vi "Configuration Tool Main.vi"() -> ()   [LabVIEW 2015, in "Configuration Tool.lvlib"]
doc: "This is the main VI for the configuration editor.Copyright 2017 National Instruments Corporation\n\nLicensed under the Apache License, Version 2.0 (the \"License\"); you may not use this file except in compliance with the License. You may obtain a copy of the License at http://www.apache.org/licenses/LICENSE-2.0\nUnless required by applicable law or agreed to in writing, software distributed under the License is distributed on an \"AS IS\" BASIS, WITHOUT WARRANTIES OR CONDITIONS OF ANY KIND, either express or implied. See the License for the specific language governing permissions and limitations under the License."
uses:
  Configuration Tool.lvlib
  Controls/StateCluster.ctl
  <vilib>/NI/Configuration Framework/Repository/NISE_CEF_Repository.lvclass
  <vilib>/NI/Configuration Framework/Node/NodeRef.ctl
  <vilib>/NI/Configuration Framework/Node/NISE_CEF_Node.lvclass
  <vilib>/NI/Configuration Framework/Node/StandardEvents.ctl
  <vilib>/NI/Configuration Framework/Node/UserEventRef.ctl
  <vilib>/NI/Configuration Framework/Controls/EventCluster.ctl
  <vilib>/NI/Configuration Framework/Node/NodeChangeEvent.ctl
  <vilib>/NI/Configuration Framework/Node/CacheState.ctl
  <vilib>/NI/Configuration Framework/Node/RefreshUIEvent.ctl
  <vilib>/NI/Configuration Framework/Node/StopEvent.ctl
  <vilib>/NI/Configuration Framework/glyph manager/glyph manager.ctl
  <vilib>/picture/picture.llb/imagedata.ctl
  Controls/StepClassLibrary.ctl
  Prototype/classes/Step/Config/Step Config.lvclass
  Controls/AddMessage.ctl
  Controls/MoveMessage.ctl
  <vilib>/Utility/error.llb/DialogType.ctl
  Classes/SequenceNode/SequenceNode.lvclass
  Classes/SequenceRepo/SequenceRepo.lvclass
  <vilib>/Utility/sysdir.llb/System Directory Type.ctl
  Classes/StepNode/StepNode.lvclass
  <vilib>/NI/AMC/Read Termination Message.vi
  <vilib>/NI/AMC/Create Single Message.vi
  <vilib>/NI/AMC/Update Message Routing Info.vi
  <vilib>/NI/AMC/Send Message.vi
  <vilib>/NI/AMC/Globals.vi
  <vilib>/NI/AMC/AMC.lvlib
  <vilib>/NI/Configuration Framework/NISE_CEF_TreeControl.lvlib
  <vilib>/NI/Configuration Framework/glyph manager/glyph manager.lvlib
panel:
  in  "View":string(tree)
  in  "Exit":bool
  # "Configurator"
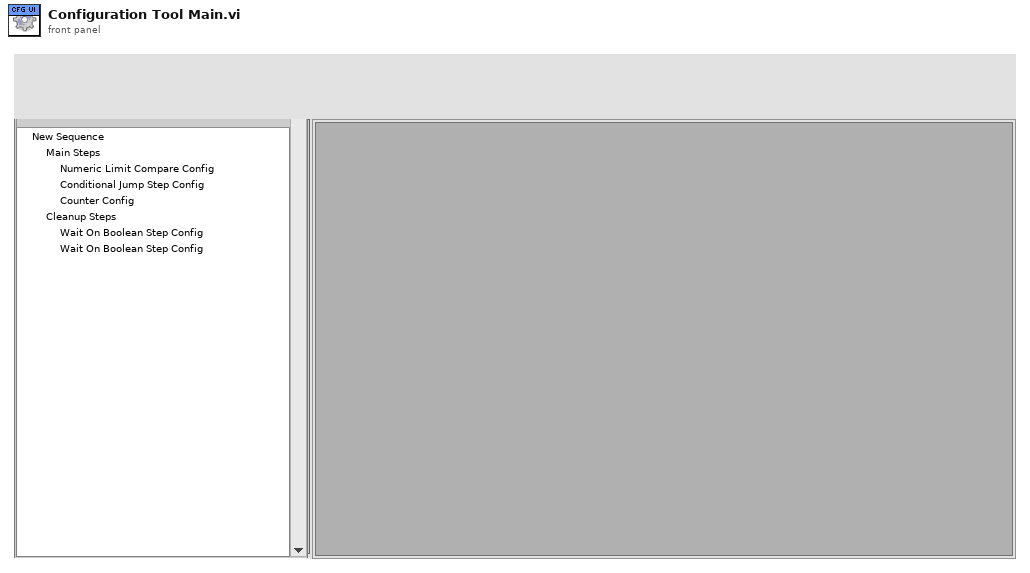
[diagram p1: front panel]
types:
  T1 = typedef "Configuration Tool.lvlib/StateCluster.ctl" = cluster{"repository":refnum<class "NISE_CEF_Repository.lvclass">, "root":T2, "unsaved changes":bool, "current path":path, "standard events":T3, "classes path":path, "glyph manager":T9, "Step Class Library":T11}
  T2 = typedef "NISE_CEF_Node.lvclass/NodeRef.ctl" = refnum<data-value>
  T3 = typedef "NISE_CEF_Node.lvclass/StandardEvents.ctl" = cluster{"user event":T4, "node change":T5, "cache state":T6, "refresh UI":T7, "stop event":T8}
  T4 = typedef "NISE_CEF_Node.lvclass/UserEventRef.ctl" = refnum<user-event>
  T5 = typedef "NISE_CEF_Node.lvclass/NodeChangeEvent.ctl" = refnum<user-event>
  T6 = typedef "NISE_CEF_Node.lvclass/CacheState.ctl" = refnum<user-event>
  T7 = typedef "NISE_CEF_Node.lvclass/RefreshUIEvent.ctl" = refnum<user-event>
  T8 = typedef "NISE_CEF_Node.lvclass/StopEvent.ctl" = refnum<user-event>
  T9 = typedef "glyph manager.lvlib/glyph manager.ctl" = cluster{"search paths":path[], "glyph map":variant, "base glyphs":T10[], "desired overlays":string[]}
  T10 = typedef "imagedata.ctl" = cluster{"image type":i32, "image depth":i32, "image":u8[], "mask":u8[], "colors":u32[], "Rectangle":cluster{"left":i16, "top":i16, "right":i16, "bottom":i16}}
  T11 = typedef "StepClassLibrary.ctl" = cluster{"Step Types":string[], "Step Config Classes":refnum<class "Step Config.lvclass">[]}
  T12 = typedef "AMC.lvlib/Message Queue.ctl" = refnum<queue>
  T13 = typedef "Configuration Tool.lvlib/AddMessage.ctl" = cluster{"node type":string, "to add to":string}
  T14 = typedef "Configuration Tool.lvlib/MoveMessage.ctl" = cluster{"node ref":T2, "new parent":T2, "Index":i32}
  T15 = typedef "Configuration Tool.lvlib/FilePaths.ctl" = cluster{"glyphs":path, "classes":path}
  T16 = typedef "DialogType.ctl" = u16
  T17 = typedef "System Directory Type.ctl" = i32
  T18 = typedef "NISE_CEF_Node.lvclass/Summary.ctl" = cluster{"ID":string, "parent ID":string, "node type":string, "text":string, "additional text":string, "glyph":string, "depth":i32, "glyph overlay":string}
  T19 = typedef "LVPoint32TypeDef.ctl" = cluster{"Horizontal":i32, "Vertical":i32}
  T20 = cluster{"data name":string, "drag data":variant}[]
  T21 = typedef "NISE_CEF_Node.lvclass/NodeMenuOptions.ctl" = cluster{"removable":bool, "movable":bool, "duplicate":bool}
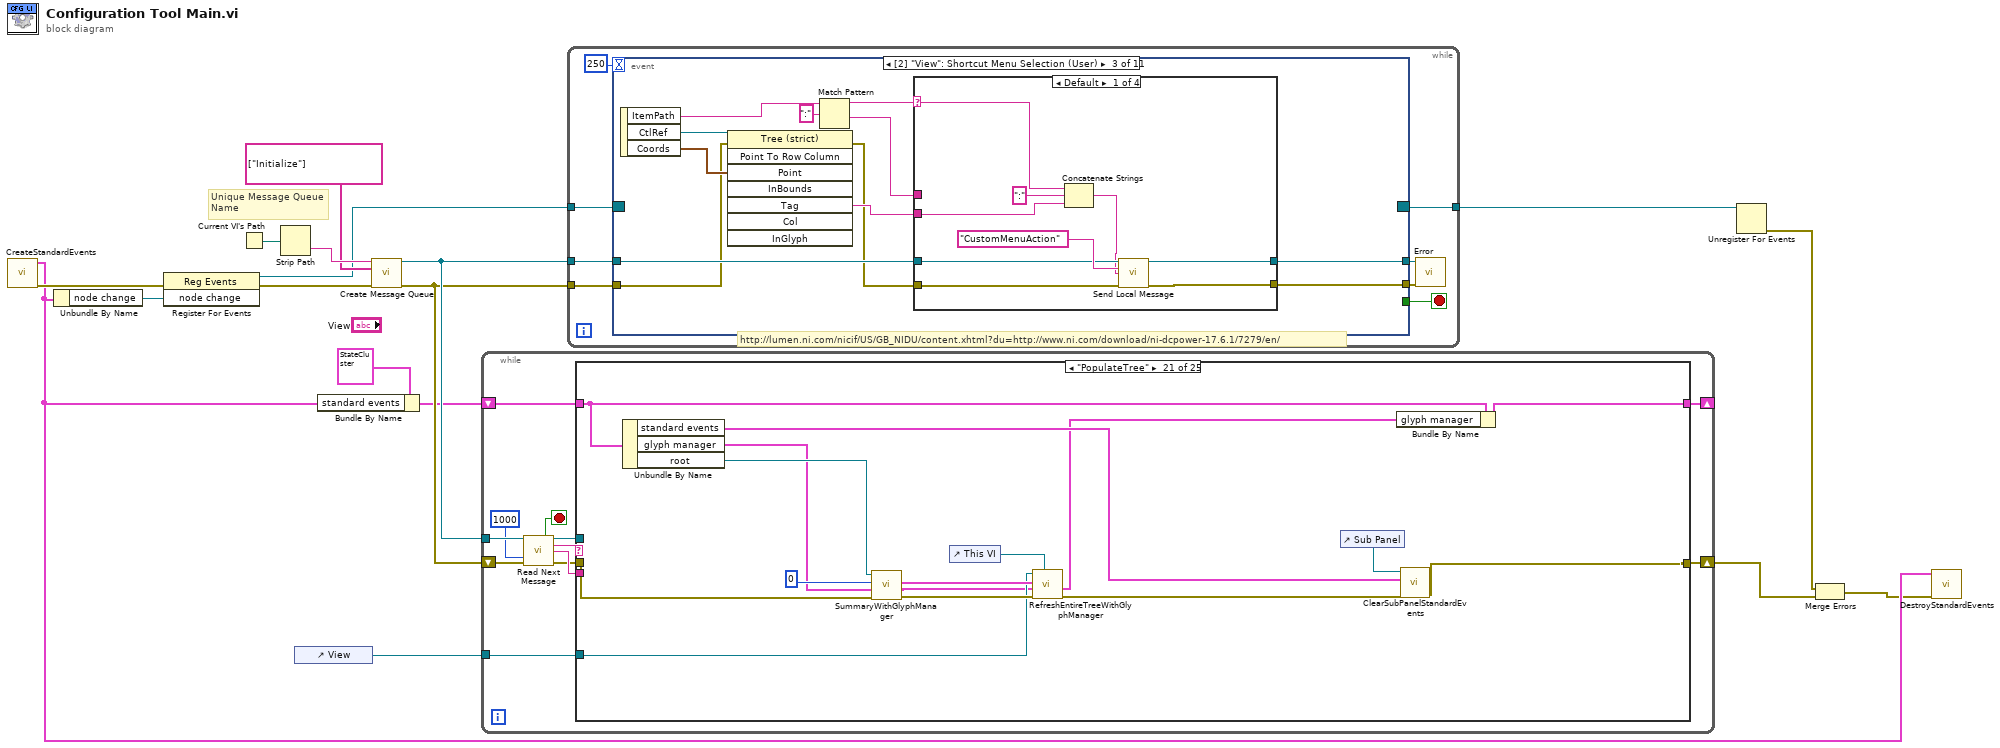
[diagram p0: block diagram]
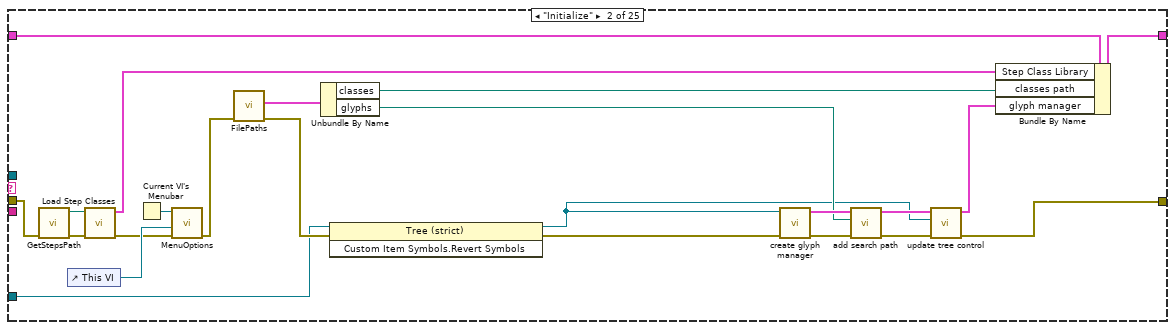
[diagram p3: hidden frame]
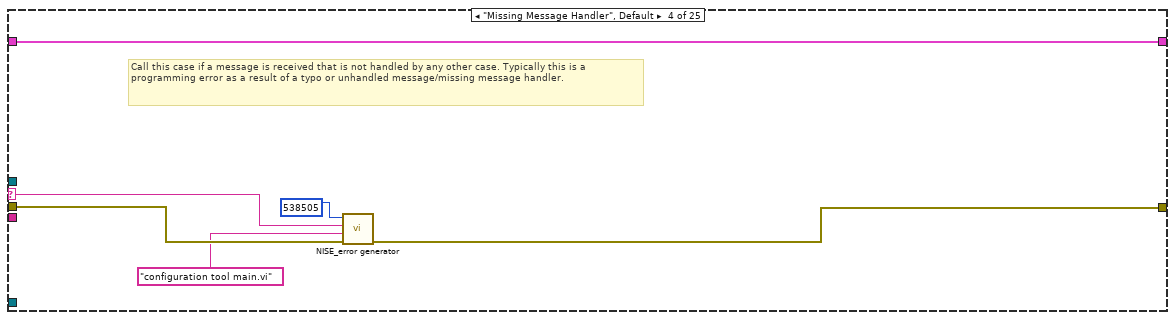
[diagram p5: hidden frame]
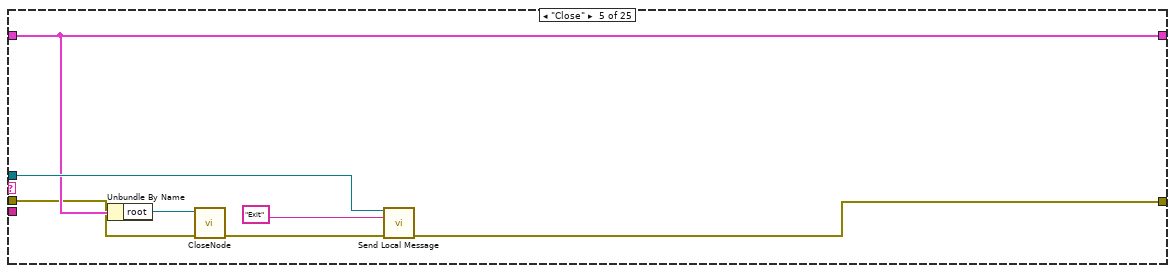
[diagram p6: hidden frame]
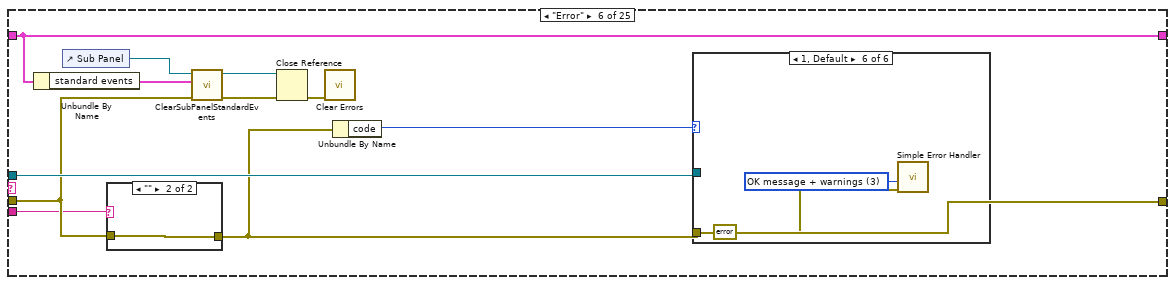
[diagram p7: hidden frame]
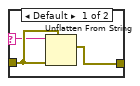
[diagram p8: hidden frame]
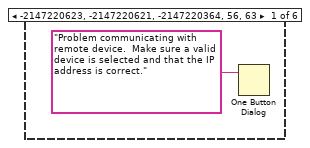
[diagram p9: hidden frame]
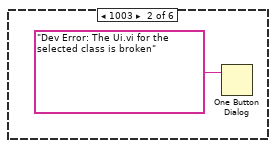
[diagram p10: hidden frame]
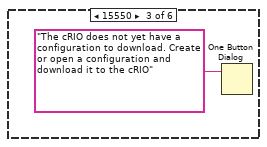
[diagram p11: hidden frame]
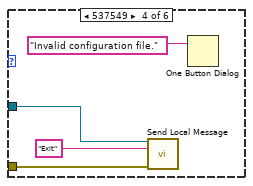
[diagram p12: hidden frame]
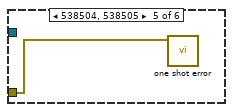
[diagram p13: hidden frame]
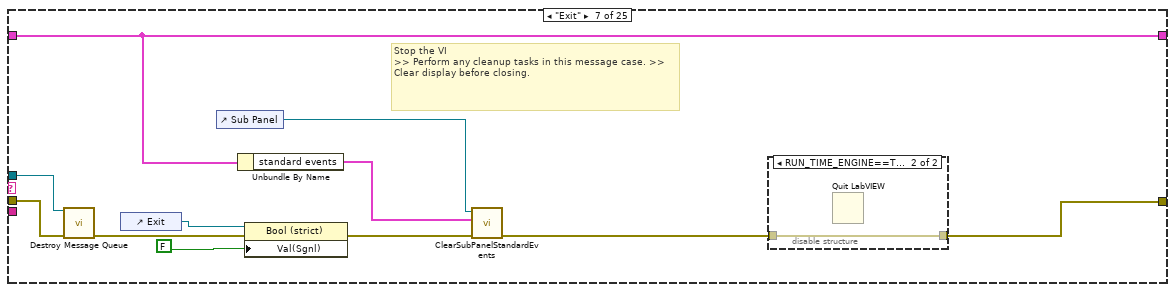
[diagram p14: hidden frame]
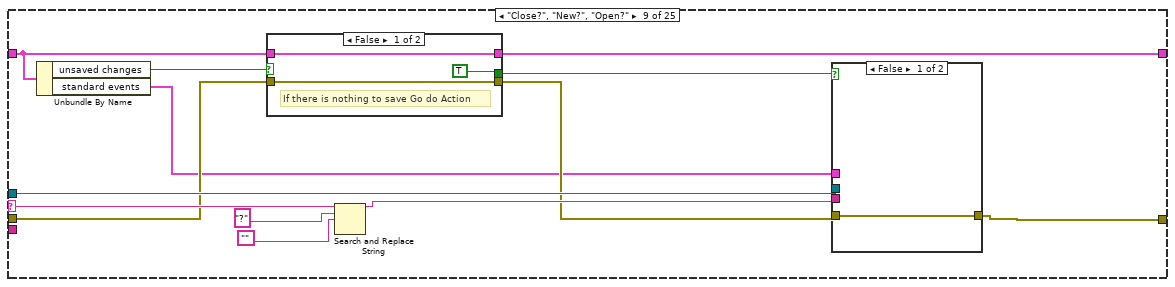
[diagram p17: hidden frame]
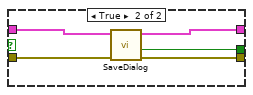
[diagram p18: hidden frame]
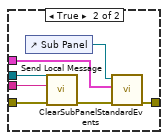
[diagram p19: hidden frame]
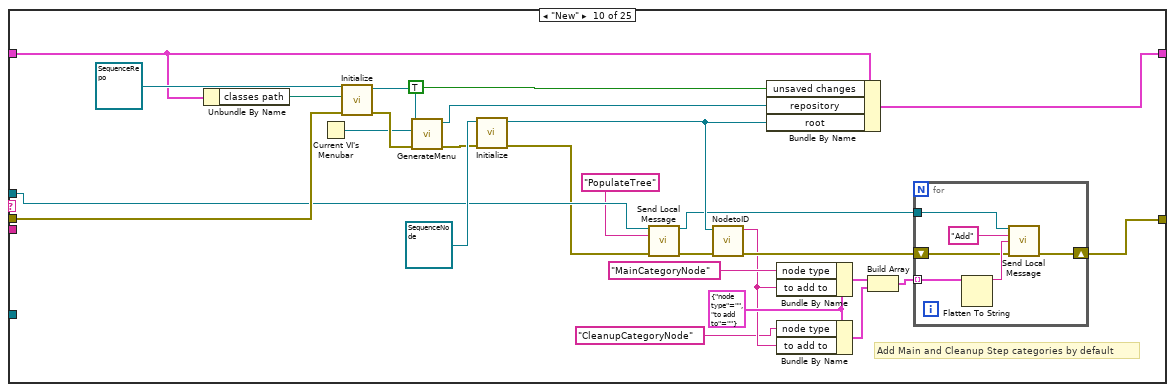
[diagram p20: hidden frame]
diagram:
  # "http://lumen.ni.com/nicif/US/GB_NIDU/content.xhtml?du=http://www.ni.com/download/ni-dcpower-17.6.1/7279/en/"
  # "Unique Message Queue Name"
  n1 = call <vilib>:"CreateStandardEvents.vi"() -> ("error out"=w12:errorcluster, "standard events"=w6:T3)  [unwired: 10 in]
  n2 = Unbundle By Name(w6) -> ("node change"=w11:T5)
  n3 = register-events(error in=w12, w11) -> (reference out=w5:refnum<event-registration>, error out=w10:errorcluster)  [unwired: 1 in]
  n4 = Current VI's Path() -> (path=w16:path)
  n5 = Strip Path(path=w16) -> (name=w17:string)  [unwired: 1 out]
  n6 = control-ref of="View"() -> (w4:refnum<vi>)
  n7 = Bundle By Name(cluster=T1 {"repository"=refnum, "root"=refnum, "unsaved changes"=FALSE, "current path"=path "", "standard events"={"user event"=refnum, "node change"=refnum, "cache state"=refnum, "refresh UI"=refnum, "stop event"=refnum}, "classes path"=path "", "glyph manager"={"search paths"=[], "glyph map"=variant, "base glyphs"=[], "desired overlays"=[]}, "Step Class Library"={"Step Types"=[], "Step Config Classes"=[]}}, "standard events"=w6) -> (w8:T1)
  n8 = call <vilib>:"Create Message Queue.vi"("message queue name"=w17, "initial message names"=string[] ["Initialize"], "error in"=w10) -> ("message queue out"=w14:T12, "error out"=w13:errorcluster)  [unwired: 11 in]
  n9 = while "Message Processor" {
    shift-right: [w25] -> w7
    shift-left: w13 -> [w24]
    tunnel: w14 -> [w23]
    shift-right: [w21] -> _
    shift-left: w8 -> [w20]
    tunnel: w4 -> [w18]
    stop <- w29 stop-if-true
    n10 = call <vilib>:"Read Next Message.vi"("message queue in"=w23, "timeout (1 ms)"=1000, "error in"=w24) -> ("exit process?"=w29:bool, "message queue out"=w19:T12, "message name"=w28:string, "message value"=w27:string, "error out"=w26:errorcluster)  [unwired: 5 in, 3 out]
    n11 = case shown="\"PopulateTree\"" w28 {
      selector: w28 -> [_ _ _ w58 _ _ _ _ w119 _ _ _ _ _ _ _ _ w352 _ _ _ _ _ _ _]
      tunnel: w27 -> [_ _ _ _ _ w71 _ _ _ _ _ _ _ w253 _ w302 w330 w350 w402 w426 _ _ w466 w487 w494]
      tunnel: w26 -> [w31 w32 w56 w61 w64 w74 w106 w110 w112 w160 w179 w219 w245 w260 w273 w294 w329 w355 w404 w425 w447 w456 w465 w485 w495]
      tunnel: [w31 w43 w56 w59 w68 errorcluster {"status"=FALSE, "code"=0, "source"=""} ("error out") w98 w110 w123 w153 w175 w223 w247 w257 w273 w296 w333 w358 w406 w422 w441 w452 w462 w480 w493] -> w25
      tunnel: [w30 w50 w55 w62 w66 w78 w97 w109 w114 w166 w180 w226 w246 w254 w272 w289 w326 w359 w405 w427 w438 w455 w460 w488 w490] -> w21
      tunnel: w20 -> [w30 w51 w55 w62 w66 w78 w97 w109 w115 w162 w181 w221 w244 w255 w272 w292 w327 w359 w397 w427 w450 w455 w460 w488 w496]
      tunnel: w19 -> [_ _ _ _ w67 w81 w105 _ w122 w151 w177 w222 _ w256 _ _ _ w353 _ _ _ _ w461 w479 w492]
      tunnel: w18 -> [_ w37 _ _ _ _ _ _ _ _ _ _ _ _ _ w290 w322 w347 w399 w420 w439 _ _ _ _]
      frame "------------Generic Operations------------" {
        # "Dummy case to add a seperation in the Case Structure menu"
      }
      frame "Initialize" {
        n12 = call "GetStepsPath.vi"("error in (no error)"=w32) -> ("error out"=w33:errorcluster, "Steps Folder Path"=w34:path)  [unwired: 9 in]
        n13 = control-ref of="This VI"() -> (w54:refnum<vi>)
        n14 = call "Load Step Classes.vi"("error in (no error)"=w33, "Step Classes Folder Path"=w34) -> ("error out"=w36:errorcluster, "Step Class Library"=w35:T11)  [unwired: 8 in]
        n15 = Current VI's Menubar() -> (w53:refnum<k9>)
        n16 = call "MenuOptions.vi"("error in"=w36, "VI ref"=w54, "menu ref in"=w53) -> ("error out"=w49:errorcluster)  [unwired: 7 in, 1 out]
        n17 = call "FilePaths.vi"("error in"=w49) -> ("error out"=w40:errorcluster, "paths"=w52:T15)  [unwired: 9 in]
        n18 = Unbundle By Name(w52) -> ("classes"=w48:path, "glyphs"=w42:path)
        n19 = invoke class="Tree (strict)" method="Custom Item Symbols.Revert Symbols"(reference=w37, error in=w40) -> (reference out=w38:refnum<vi>, error out=w39:errorcluster)  [unwired: 1 in, 1 out]
        n20 = call <vilib>:"create glyph manager.vi"("error in"=w39, "tree ref (for default symbols)"=w38) -> ("error out"=w47:errorcluster, "glyph manager"=w46:T9)  [unwired: 8 in]
        n21 = call <vilib>:"add search path.vi"("error in"=w47, "search path"=w42, "glyph manager in"=w46) -> ("error out"=w45:errorcluster, "glyph manager out"=w44:T9)  [unwired: 7 in]
        n22 = call <vilib>:"update tree control.vi"("error in"=w45, "tree reference"=w38, "glyph manager in"=w44) -> ("error out"=w43:errorcluster, "glyph manager out"=w41:T9)  [unwired: 7 in]
        n23 = Bundle By Name(cluster=w51, "Step Class Library"=w35, "classes path"=w48, "glyph manager"=w41) -> (w50:T1)
      }
      frame "", "Idle" {
      }
      frame "Missing Message Handler", Default {
        # "Call this case if a message is received that is not handled by any other case. Typically this is a programming error as a result of a typo or unhandled message/missing message handler."
        n24 = call <vilib>:"NISE_error generator.vi"("error in"=w61, "source"="configuration tool main.vi", "append error message"=w58, "error code (0)"=538505) -> ("error out"=w59:errorcluster)  [unwired: 5 in]
      }
      frame "Close" {
        n25 = Unbundle By Name(w66) -> ("root"=w65:T2)
        n26 = call <vilib>:"CloseNode.vi"("error in"=w64, "node ref"=w65) -> ("error out"=w63:errorcluster)  [unwired: 9 in]
        n27 = call <vilib>:"Send Local Message.vi"("message queue in"=w67, "message name"="Exit", "error in"=w63) -> ("error out"=w68:errorcluster)  [unwired: 10 in, 2 out]
      }
      frame "Error" {
        n28 = Unbundle By Name(w78) -> ("standard events"=w70:T3)
        n29 = control-ref of="Sub Panel"() -> (w77:refnum<vi>)
        n30 = case shown="\"\"" w71 {
          selector: w71 -> [w83 _]
          tunnel: w74 -> [w84 w85]
          tunnel: [w82 w85] -> w73
          frame Default {
            n31 = Unflatten From String(type=w84, binary string=w83, error in (no error)=w84) -> (value=w82:errorcluster)  [unwired: 2 in, 2 out]
          }
          frame "" {
          }
        }
        n32 = call <vilib>:"ClearSubPanelStandardEvents.vi"("error in"=w74, "standard events"=w70, "sub panel ref in"=w77) -> ("error out"=w76:errorcluster, "sub panel ref out"=w75:refnum<vi>)  [unwired: 7 in]
        n33 = Close Reference(reference=w75, error in (no error)=w76) -> (error out=w72:errorcluster)
        n34 = call <vilib>:"Clear Errors.vi"("error in (no error)"=w72) -> ()  [unwired: 5 in, 2 out]
        n35 = Unbundle By Name(w73) -> ("code"=w79:i32)
        n36 = case shown="1, Default" w79 {
          tunnel: w81 -> [_ _ _ w91 _ _]
          tunnel: w73 -> [_ _ _ w90 w93 w95]
          frame -2147220623, -2147220621, -2147220364, 56, 63 {
            n37 = One Button Dialog(message="Problem communicating with remote device.  Make sure a valid device is selected and that the IP address is correct.") -> ()  [unwired: 1 in, 1 out]
          }
          frame 1003 {
            n38 = One Button Dialog(message="Dev Error: The Ui.vi for the selected class is broken") -> ()  [unwired: 1 in, 1 out]
          }
          frame 15550 {
            n39 = One Button Dialog(message="The cRIO does not yet have a configuration to download. Create or open a configuration and download it to the cRIO") -> ()  [unwired: 1 in, 1 out]
          }
          frame 537549 {
            n40 = call <vilib>:"Send Local Message.vi"("message queue in"=w91, "message name"="Exit", "error in"=w90) -> ()  [unwired: 10 in, 3 out]
            n41 = One Button Dialog(message="Invalid configuration file.") -> ()  [unwired: 1 in, 1 out]
          }
          frame 538504, 538505 {
            n42 = call <vilib>:"one shot error.vi"("error in"=w93) -> ()  [unwired: 11 in]
          }
          frame 1, Default {
            w94 = T16 3 items=["no dialog", "OK message", "continue or stop message", "OK message + warnings", "continue/stop + warnings"] ("type of dialog (OK msg:1)")
            n43 = call <vilib>:"Simple Error Handler.vi"("type of dialog (OK msg:1)"=w94, "error in (no error)"=w95) -> ()  [unwired: 8 out]
          }
        }
      }
      frame "Exit" {
        # "Stop the VI                                                                             >> Perform any cleanup tasks in this message case. >> Clear display before closing."
        n44 = call <vilib>:"Destroy Message Queue.vi"("message queue in"=w105, "error in"=w106) -> ("error out"=w102:errorcluster)  [unwired: 11 in, 2 out]
        n45 = control-ref of="Exit"() -> (w104:refnum<vi>)
        n46 = control-ref of="Sub Panel"() -> (w101:refnum<vi>)
        n47 = Unbundle By Name(w97) -> ("standard events"=w96:T3)
        n48 = property class="Bool (strict)"(reference=w104, error in=w102, "Val(Sgnl)"=FALSE ("Exit")) -> (error out=w100:errorcluster)  [unwired: 1 out]
        n49 = call <vilib>:"ClearSubPanelStandardEvents.vi"("error in"=w100, "standard events"=w96, "sub panel ref in"=w101) -> ("error out"=w99:errorcluster)  [unwired: 7 in, 1 out]
        n50 = disable-structure shown="RUN_TIME_ENGINE==True" {
          disable-tunnel: [w107 w108] -> w98
          disable-tunnel: w99 -> [w107 w108]
          frame condition #0 (active) {
          }
          frame condition #1 {
            n51 = Quit LabVIEW() -> ()  [unwired: 1 in]
          }
        }
      }
      frame "------------Menu Operations--------------" {
        # "Dummy case to add a seperation in the Case Structure menu"
      }
      frame "Close?", "New?", "Open?" {
        n52 = Unbundle By Name(w115) -> ("unsaved changes"=w117:bool, "standard events"=w111:T3)
        n53 = case shown="False" w117 {
          tunnel: [TRUE ("SaveFlag") w131] -> w116
          tunnel: w115 -> [w125 w130]
          tunnel: [w125 w129] -> w114
          tunnel: w112 -> [w124 w128]
          tunnel: [w124 w127] -> w113
          frame False {
            # "If there is nothing to save Go do Action"
          }
          frame True {
            n54 = call "SaveDialog.vi"("error in"=w128, "state in"=w130) -> ("error out"=w127:errorcluster, "new"=w131:bool, "state out"=w129:T1)  [unwired: 7 in]
          }
        }
        n55 = Search and Replace String(input string=w119, search string="?", replace string="") -> (result string=w118:string)  [unwired: 5 in, 3 out]
        n56 = case shown="False" w116 {
          tunnel: w113 -> [w132 w139]
          tunnel: [w132 w135] -> w123
          tunnel: w122 -> [_ w138]
          tunnel: w118 -> [_ w137]
          tunnel: w111 -> [_ w133]
          frame False {
          }
          frame True {
            n57 = control-ref of="Sub Panel"() -> (w134:refnum<vi>)
            n58 = call <vilib>:"Send Local Message.vi"("message queue in"=w138, "message name"=w137, "error in"=w139) -> ("error out"=w136:errorcluster)  [unwired: 10 in, 2 out]
            n59 = call <vilib>:"ClearSubPanelStandardEvents.vi"("error in"=w136, "standard events"=w133, "sub panel ref in"=w134) -> ("error out"=w135:errorcluster)  [unwired: 7 in, 1 out]
          }
        }
      }
      frame "New" {
        w143 = T13 {"node type"="", "to add to"=""} ("input cluster")
        # "Add Main and Cleanup Step categories by default"
        n60 = Unbundle By Name(w162) -> ("classes path"=w161:path)
        n61 = Current VI's Menubar() -> (w155:refnum<k9>)
        n62 = call-dynamic "Initialize.vi"("error in"=w160, "path"=w161, "repository in"=refnum<class "SequenceRepo.lvclass"> refnum ("cRIORepo.lvclass")) -> ("error out"=w159:errorcluster, "repository out"=w157:refnum<class "SequenceRepo.lvclass">)  [unwired: 7 in]
        n63 = call-dynamic "GenerateMenu.vi"("error in"=w159, "menu ref in"=w155, "NISE_CEF_Repository in"=w157) -> ("error out"=w158:errorcluster, "NISE_CEF_Repository out"=w156:refnum<class "SequenceRepo.lvclass">)  [unwired: 6 in, 1 out]
        n64 = call-dynamic "Initialize.vi"("error in"=w158, "SequenceNode in"=refnum<class "SequenceNode.lvclass"> refnum ("cRIO.lvclass")) -> ("error out"=w148:errorcluster, "data value reference"=w154:T2)  [unwired: 7 in, 1 out]
        n65 = call <vilib>:"Send Local Message.vi"("message queue in"=w151, "message name"="PopulateTree", "error in"=w148) -> ("message queue out"=w150:T12, "error out"=w147:errorcluster)  [unwired: 10 in, 1 out]
        n66 = call <vilib>:"NodetoID.vi"("error in"=w147, "node ref"=w154) -> ("error out"=w146:errorcluster, "ID"=w141:string)  [unwired: 8 in]
        n67 = Bundle By Name(cluster=w162, "unsaved changes"=TRUE ("SaveFlag"), "repository"=w156, "root"=w154) -> (w166:T1)
        n68 = Bundle By Name(cluster=w143, "node type"="MainCategoryNode", "to add to"=w141) -> (w144:T13)
        n69 = Bundle By Name(cluster=w143, "node type"="CleanupCategoryNode", "to add to"=w141) -> (w142:T13)
        n70 = Build Array(w144, w142) -> (w145:T13[])
        n71 = for {
          tunnel: w145 -> [w170] mode=indexing
          tunnel: w150 -> [w168]
          shift-right: [w172] -> w153
          shift-left: w146 -> [w167]
          n72 = Flatten To String(anything=w170) -> (data string=w169:string)  [unwired: 3 in, 2 out]
          n73 = call <vilib>:"Send Local Message.vi"("message queue in"=w168, "message name"="Add", "message value"=w169, "error in"=w167) -> ("error out"=w172:errorcluster)  [unwired: 9 in, 2 out]
        }
      }
      frame "Open" {
        w174 = T17 0 items=["User Home"=0, "User Desktop"=1, "User Documents"=2, "User Application Data"=3, "User Preferences"=4, "User Temporary"=5, "Public Documents"=6, "Public Application Data"=7, "Public Preferences"=8, "Public Cache"=13, "System Core Libraries"=9, "System Installed Libraries"=10, "Application Files"=11, "Boot Volume Root"=12] ("system directory type")
        n74 = call <vilib>:"Get System Directory.vi"("system directory type"=w174) -> ("system directory"=w173:path)  [unwired: 10 in]
        n75 = in-place {
          in-place-border: w179 -> [w187]
          in-place-border: [w186] -> w176
          in-place-border: w173 -> [w182]
          n76 = in-place-cluster #1(w181) -> ("current path"=w184:path, "repository"=w195:refnum<class "NISE_CEF_Repository.lvclass">, "root"=w191:T2)  [unwired: 1 out]
          n77 = call "FileDialog.vi"("error in"=w187, "start path"=w182) -> ("error out"=w188:errorcluster, "cancelled"=w189:bool, "selected path"=w185:path)  [unwired: 7 in]
          n78 = Compound Arithmetic op=OR(invert w189) -> (w190:bool)
          n79 = case shown="True" w190 {
            tunnel: w195 -> [w196 w208]
            tunnel: [w196 w206] -> w193
            tunnel: [w197 w204] -> w186
            tunnel: [w198 w203] -> w192
            tunnel: w185 -> [_ w201]
            tunnel: w188 -> [w197 w200]
            tunnel: w191 -> [w198 w199]
            frame False {
            }
            frame True {
              n80 = call-dynamic "Open.vi"("error in"=w200, "file path"=w201, "repository in"=w208) -> ("error out"=w205:errorcluster, "invalid?"=w202:bool, "repository out"=w207:refnum<class "NISE_CEF_Repository.lvclass">)  [unwired: 6 in]
              n81 = case shown="False" w202 {
                tunnel: w207 -> [w213 w216]
                tunnel: [w212 w216] -> w206
                tunnel: w205 -> [w211 w215]
                tunnel: [w210 w215] -> w204
                tunnel: [w209 w214] -> w203
                tunnel: w199 -> [_ w214]
                frame False {
                  n82 = call-dynamic "WriteTree.vi"("error in"=w211, "repository in"=w213) -> ("error out"=w210:errorcluster, "root"=w209:T2, "repository out"=w212:refnum<class "NISE_CEF_Repository.lvclass">)  [unwired: 7 in]
                }
                frame True {
                }
              }
            }
          }
          n83 = Select(t=w184, s=w186, f=w185) -> (s? t:f=w183:path)
          n84 = in-place-cluster #1("current path"=w183, "unsaved changes"=FALSE ("SaveFlag"), "repository"=w193, "root"=w192) -> (w180:T1)
        }
        n85 = call <vilib>:"Send Local Message.vi"("message queue in"=w177, "message name"="PopulateTree", "error in"=w176) -> ("error out"=w175:errorcluster)  [unwired: 10 in, 2 out]
      }
      frame "Save" {
        n86 = in-place {
          in-place-border: w219 -> [w230]
          in-place-border: [w229] -> w218
          in-place-border: [w227] -> w217
          n87 = in-place-cluster #2(w221) -> ("current path"=w228:path, "root"=w231:T2, "repository"=w233:refnum<class "NISE_CEF_Repository.lvclass">)
          n88 = Empty String/Path?(string/path=w228) -> (empty?=w227:bool)
          n89 = call-dynamic "ReadTree.vi"("error in"=w230, "root"=w231, "repository in"=w233) -> ("error out"=w229:errorcluster, "repository out"=w232:refnum<class "NISE_CEF_Repository.lvclass">)  [unwired: 7 in]
          n90 = in-place-cluster #2("current path"=w228, "root"=w231, "repository"=w232) -> (w220:T1)
        }
        n91 = case shown="True" w217 {
          tunnel: w220 -> [w237 w239]
          tunnel: [w236 w238] -> w226
          tunnel: [w235 w240] -> w224
          tunnel: w218 -> [w234 w241]
          frame False {
            n92 = call "Save.vi"("error in"=w234, "state in"=w237) -> ("error out"=w235:errorcluster, "state out"=w236:T1)  [unwired: 8 in]
          }
          frame True {
            # "Empty path use Dialog"
            n93 = call "SaveAs.vi"("error in"=w241, "state in"=w239) -> ("error out"=w240:errorcluster, "state out"=w238:T1)  [unwired: 7 in, 1 out]
          }
        }
        n94 = call <vilib>:"Send Local Message.vi"("message queue in"=w222, "message name"="PopulateTree", "error in"=w224) -> ("error out"=w223:errorcluster)  [unwired: 10 in, 2 out]
      }
      frame "SaveAs" {
        n95 = in-place {
          in-place-border: w245 -> [w249]
          in-place-border: [w248] -> w243
          n96 = in-place-cluster #3(w244) -> ("root"=w250:T2, "repository"=w252:refnum<class "NISE_CEF_Repository.lvclass">)
          n97 = call-dynamic "ReadTree.vi"("error in"=w249, "root"=w250, "repository in"=w252) -> ("error out"=w248:errorcluster, "repository out"=w251:refnum<class "NISE_CEF_Repository.lvclass">)  [unwired: 7 in]
          n98 = in-place-cluster #3("root"=w250, "repository"=w251) -> (w242:T1)
        }
        n99 = call "SaveAs.vi"("error in"=w243, "state in"=w242) -> ("error out"=w247:errorcluster, "state out"=w246:T1)  [unwired: 7 in, 1 out]
      }
      frame "Custom View" {
        n100 = in-place {
          in-place-border: w260 -> [w271]
          in-place-border: [w270] -> w258
          in-place-border: w253 -> [w261]
          n101 = in-place-cluster #4(w255) -> ("repository"=w265:refnum<class "NISE_CEF_Repository.lvclass">, "root"=w264:T2)
          n102 = call-dynamic "ReadTree.vi"("error in"=w271, "root"=w264, "repository in"=w265) -> ("error out"=w268:errorcluster, "repository out"=w267:refnum<class "NISE_CEF_Repository.lvclass">)  [unwired: 7 in]
          n103 = call-dynamic "CustomView.vi"("error in"=w268, "view name"=w261, "repository in"=w267) -> ("error out"=w269:errorcluster, "repository out"=w266:refnum<class "NISE_CEF_Repository.lvclass">)  [unwired: 7 in]
          n104 = call-dynamic "WriteTree.vi"("error in"=w269, "repository in"=w266) -> ("error out"=w270:errorcluster, "root"=w262:T2, "repository out"=w263:refnum<class "NISE_CEF_Repository.lvclass">)  [unwired: 7 in]
          n105 = in-place-cluster #4("repository"=w263, "root"=w262) -> (w254:T1)
        }
        n106 = call <vilib>:"Send Local Message.vi"("message queue in"=w256, "message name"="PopulateTree", "error in"=w258) -> ("error out"=w257:errorcluster)  [unwired: 10 in, 2 out]
      }
      frame "-------TreeControl Operations-----------" {
        # "Dummy case to add a seperation in the Case Structure menu"
      }
      frame "Add" {
        n107 = Unflatten From String(type=T13 {"node type"="", "to add to"=""} ("input cluster"), binary string=w302) -> (value=w300:T13)  [unwired: 3 in, 2 out]
        n108 = Unbundle By Name(w300) -> ("to add to"=w298:string, "node type"=w281:string)
        n109 = Match Pattern(string=w281, regular expression=":") -> (before substring=w280:string, after substring=w279:string)  [unwired: 1 in, 2 out]
        n110 = in-place {
          in-place-border: w294 -> [w319]
          in-place-border: [w318] -> w293
          in-place-border: [w317] -> w291
          in-place-border: w280 -> [w316]
          n111 = in-place-cluster #5(w292) -> ("repository"=w321:refnum<class "NISE_CEF_Repository.lvclass">)
          n112 = call-dynamic "GetClassPath.vi"("error in"=w319, "class name"=w316, "Repository in"=w321) -> ("error out"=w318:errorcluster, "class path"=w317:path, "Repository out"=w320:refnum<class "NISE_CEF_Repository.lvclass">)  [unwired: 6 in]
          n113 = in-place-cluster #5("repository"=w320) -> (w275:T1)
        }
        n114 = Unbundle By Name(w275) -> ("glyph manager"=w287:T9)
        n115 = Unbundle By Name(w275) -> ("Step Class Library"=w274:T11)
        n116 = call <vilib>:"Get LV Class Default Value.vi"("error in (no error)"=w293, "class path"=w291) -> ("error out"=w303:errorcluster, "object"=w304:refnum<class>)  [unwired: 8 in]
        n117 = To More Specific Class(target class=refnum<class "NISE_CEF_Node.lvclass"> refnum ("Node.lvclass"), reference=w304, error in=w303) -> (specific class reference=w276:refnum<class "NISE_CEF_Node.lvclass">, error out=w288:errorcluster)
        n118 = case shown="Default" w279 {
          selector: w279 -> [_ w309]
          tunnel: w288 -> [w306 w315]
          tunnel: [w306 w314] -> w278
          tunnel: [w305 w313] -> w277
          tunnel: w276 -> [w305 w311]
          tunnel: w274 -> [_ w307]
          frame "" {
          }
          frame Default {
            n119 = To More Specific Class(target class=refnum<class "StepNode.lvclass"> refnum ("StepNode.lvclass"), reference=w311, error in=w315) -> (specific class reference=w310:refnum<class "StepNode.lvclass">, error out=w312:errorcluster)
            n120 = call-dynamic "LoadStepType.vi"("error in (no error)"=w312, "Step Type Class Element"=w307, "Step Type"=w309, "StepNode in"=w310) -> ("error out"=w314:errorcluster, "StepNode out"=w313:refnum<class "StepNode.lvclass">)  [unwired: 6 in]
          }
        }
        n121 = call-dynamic "AddGlyphtoGManager.vi"("error in"=w278, "glyph manager"=w287, "NISE_CEF_Node in"=w277) -> ("error out"=w285:errorcluster, "glyph manager out"=w286:T9, "NISE_CEF_Node out"=w284:refnum<class "NISE_CEF_Node.lvclass">)  [unwired: 6 in]
        n122 = call <vilib>:"AddNode.vi"("error in"=w285, "node in"=w284, "parent node ID"=w298) -> ("error out"=w297:errorcluster, "summary"=w295:T18[])  [unwired: 7 in]
        n123 = call <vilib>:"PopulateTreeSumaryWithGlyphManager.vi"("error in"=w297, "glyph manager"=w286, "summary"=w295, "tree ref in"=w290) -> ("error out"=w296:errorcluster, "glyph manager out"=w283:T9)  [unwired: 6 in]
        n124 = Bundle By Name(cluster=w275, "glyph manager"=w283) -> (w289:T1)
      }
      frame "Duplicate" {
        n125 = call <vilib>:"IDtoNode.vi"("error in"=w329, "ID"=w330) -> ("error out"=w331:errorcluster, "invalid Id"=w328:bool, "node ref"=w332:T2)  [unwired: 7 in]
        n126 = Unbundle By Name(w327) -> ("glyph manager"=w324:T9)
        n127 = case shown="False" w328 {
          tunnel: [w344 w346] -> w333
          tunnel: w332 -> [w343 _]
          tunnel: w331 -> [w340 w346]
          tunnel: w324 -> [w336 w345]
          tunnel: [w335 w345] -> w323
          tunnel: w322 -> [w334 _]
          frame False {
            n128 = call <vilib>:"DuplicateNode.vi"("same parent?"=TRUE ("s"), "error in"=w340, "node ref in"=w343) -> ("error out"=w341:errorcluster, "new node ref"=w342:T2)  [unwired: 7 in]
            n129 = call <vilib>:"Summary.vi"("error in"=w341, "node self ref"=w342) -> ("error out"=w338:errorcluster, "summary"=w337:T18[])  [unwired: 8 in]
            n130 = call <vilib>:"PopulateTreeSumaryWithGlyphManager.vi"("error in"=w338, "glyph manager"=w336, "summary"=w337, "tree ref in"=w334) -> ("error out"=w344:errorcluster, "glyph manager out"=w335:T9)  [unwired: 6 in]
          }
          frame True {
          }
        }
        n131 = Bundle By Name(cluster=w327, "unsaved changes"=TRUE, "glyph manager"=w323) -> (w326:T1)
      }
      frame "CustomMenuAction" {
        n132 = Match Pattern(string=w350, regular expression=":") -> (before substring=w349:string, after substring=w348:string)  [unwired: 1 in, 2 out]
        n133 = call <vilib>:"IDtoNode.vi"("error in"=w355, "ID"=w348) -> ("error out"=w356:errorcluster, "invalid Id"=w354:bool, "node ref"=w357:T2)  [unwired: 7 in]
        n134 = case shown="False" w354 {
          tunnel: [w365 w395] -> w358
          tunnel: w357 -> [w362 _]
          tunnel: w356 -> [w368 w395]
          tunnel: w353 -> [w369 _]
          tunnel: w352 -> [_ _]
          tunnel: w349 -> [w366 _]
          tunnel: w347 -> [w363 _]
          frame False {
            n135 = in-place {
              in-place-border: w369 -> [w393]
              in-place-border: w368 -> [w391]
              in-place-border: [w390] -> w364
              in-place-border: [w389] -> w367
              in-place-border: w366 -> [w388]
              in-place-border: w363 -> [w387]
              in-place-border: [w386] -> w361
              n136 = in-place-dvr #6(w362) -> (w394:refnum<class "NISE_CEF_Node.lvclass">)  [unwired: 1 out]
              n137 = call-dynamic "MenuHandler.vi"("tree control"=w387, "main message queue"=w393, "error in"=w391, "menu string"=w388, "NISE_CEF_Node in"=w394) -> ("error out"=w390:errorcluster, "refresh tree?"=w386:bool, "Unhandled"=w389:bool, "NISE_CEF_Node out"=w392:refnum<class "NISE_CEF_Node.lvclass">)  [unwired: 3 in]
              n138 = in-place-dvr #6(w392) -> (w360:T2)  [unwired: 1 out]
            }
            n139 = case shown="False" w367 {
              tunnel: w366 -> [_ w381]
              tunnel: [w373 w382] -> w365
              tunnel: w364 -> [w371 w383]
              tunnel: w361 -> [w370 _]
              tunnel: w360 -> [w372 _]
              frame False {
                n140 = case shown="True" w370 {
                  tunnel: [w374 w377] -> w373
                  tunnel: w372 -> [_ w376]
                  tunnel: w371 -> [w374 w375]
                  frame False {
                  }
                  frame True {
                    n141 = call <vilib>:"NodetoID.vi"("error in"=w375, "node ref"=w376) -> ("error out"=w379:errorcluster, "ID"=w380:string)  [unwired: 8 in]
                    n142 = call <vilib>:"Send Local Message.vi"("message name"="NodeDataChange", "message value"=w380, "error in"=w379) -> ("error out"=w377:errorcluster)  [unwired: 10 in, 2 out]
                  }
                }
              }
              frame True {
                n143 = call <vilib>:"NISE_error generator.vi"("error in"=w383, "source"="configuration tool main.vi", "append error message"=w381, "error code (0)"=538506) -> ("error out"=w382:errorcluster)  [unwired: 5 in]
              }
            }
          }
          frame True {
          }
        }
      }
      frame "RefreshNode" {
        # "Refreshes the node in the Tree, Sets the save flag to true. This case can be called from the UIs of the nodes"
        n144 = Unbundle By Name(w397) -> ("glyph manager"=w396:T9)
        n145 = call <vilib>:"IDtoNode.vi"("error in"=w404, "ID"=w402) -> ("error out"=w403:errorcluster, "invalid Id"=w400:bool, "node ref"=w401:T2)  [unwired: 7 in]
        n146 = case shown="False" w400 {
          tunnel: [w416 w419] -> w406
          tunnel: w403 -> [w412 w419]
          tunnel: w401 -> [w411 _]
          tunnel: w399 -> [w410 _]
          tunnel: [w409 w418] -> w398
          tunnel: w396 -> [w407 w418]
          frame False {
            n147 = call <vilib>:"SummaryWithGlyphManager.vi"("error in"=w412, "glyph manager"=w407, "node self ref"=w411) -> ("error out"=w414:errorcluster, "glyph manager out"=w408:T9, "summary"=w413:T18[])  [unwired: 6 in]
            n148 = call <vilib>:"RefreshSubTreeWithGlyphManager.vi"("error in"=w414, "glyph manager"=w408, "node information"=w413, "tree ref in"=w410) -> ("error out"=w417:errorcluster, "glyph manager out"=w409:T9, "tree ref out"=w415:refnum<vi>)  [unwired: 5 in]
            n149 = Close Reference(reference=w415, error in (no error)=w417) -> (error out=w416:errorcluster)
          }
          frame True {
          }
        }
        n150 = Bundle By Name(cluster=w397, "glyph manager"=w398) -> (w405:T1)
      }
      frame "RemoveNode" {
        n151 = call <vilib>:"IDtoNode.vi"("error in"=w425, "ID"=w426) -> ("error out"=w424:errorcluster, "invalid Id"=w421:bool, "node ref"=w423:T2)  [unwired: 7 in]
        n152 = case shown="False" w421 {
          tunnel: w424 -> [w433 w434]
          tunnel: w423 -> [w432 _]
          tunnel: [w429 w434] -> w422
          tunnel: w420 -> [w428 _]
          frame False {
            n153 = call <vilib>:"RemoveNode.vi"("error in"=w433, "node"=w432) -> ("error out"=w430:errorcluster, "node ID"=w431:string)  [unwired: 8 in]
            n154 = call <vilib>:"ClearTreeNode.vi"("error in"=w430, "tag"=w431, "tree reference"=w428) -> ("error out"=w429:errorcluster)  [unwired: 8 in]
          }
          frame True {
          }
        }
      }
      frame "PopulateTree" {
        n155 = Unbundle By Name(w450) -> ("standard events"=w440:T3, "glyph manager"=w436:T9, "root"=w445:T2)
        n156 = call <vilib>:"SummaryWithGlyphManager.vi"("error in"=w447, "glyph manager"=w436, "depth"=0 ("Depth"), "node self ref"=w445) -> ("error out"=w446:errorcluster, "glyph manager out"=w435:T9, "summary"=w449:T18[])  [unwired: 5 in]
        n157 = control-ref of="This VI"() -> (w448:refnum<vi>)
        n158 = call <vilib>:"RefreshEntireTreeWithGlyphManager.vi"("calling VI in"=w448, "error in"=w446, "glyph manager"=w435, "array"=w449, "tree ref in"=w439) -> ("error out"=w442:errorcluster, "glyph manager out"=w437:T9)  [unwired: 5 in]
        n159 = control-ref of="Sub Panel"() -> (w443:refnum<vi>)
        n160 = Bundle By Name(cluster=w450, "glyph manager"=w437) -> (w438:T1)
        n161 = call <vilib>:"ClearSubPanelStandardEvents.vi"("error in"=w442, "standard events"=w440, "sub panel ref in"=w443) -> ("error out"=w441:errorcluster)  [unwired: 7 in, 1 out]
      }
      frame "CleansubPanel" {
        n162 = Unbundle By Name(w455) -> ("standard events"=w451:T3)
        n163 = control-ref of="Sub Panel"() -> (w457:refnum<vi>)
        n164 = call <vilib>:"ClearSubPanelStandardEvents.vi"("error in"=w456, "standard events"=w451, "sub panel ref in"=w457) -> ("error out"=w454:errorcluster, "sub panel ref out"=w453:refnum<vi>)  [unwired: 7 in]
        n165 = Close Reference(reference=w453, error in (no error)=w454) -> (error out=w452:errorcluster)
      }
      frame "ActivateNode" {
        n166 = Unbundle By Name(w460) -> ("standard events"=w459:T3)
        n167 = call <vilib>:"IDtoNode.vi"("error in"=w465, "ID"=w466) -> ("error out"=w458:errorcluster, "invalid Id"=w464:bool, "node ref"=w463:T2)  [unwired: 7 in]
        n168 = case shown="False" w464 {
          tunnel: w463 -> [w473 _]
          tunnel: [w474 w475] -> w462
          tunnel: w458 -> [w471 w475]
          tunnel: w461 -> [w469 _]
          tunnel: w459 -> [w467 _]
          frame False {
            n169 = control-ref of="Sub Panel"() -> (w470:refnum<vi>)
            n170 = call <vilib>:"ClearSubPanelStandardEvents.vi"("error in"=w471, "standard events"=w467, "sub panel ref in"=w470) -> ("error out"=w472:errorcluster, "sub panel ref out"=w468:refnum<vi>)  [unwired: 7 in]
            n171 = call <vilib>:"LoadNodeUIStandardEvents.vi"("user event out"=w467, "error in"=w472, "sub panel ref in"=w468, "main queue"=w469, "node"=w473) -> ("error out"=w474:errorcluster)  [unwired: 6 in]
          }
          frame True {
          }
        }
      }
      frame "Move" {
        n172 = Unflatten From String(type=T14 {"node ref"=refnum, "new parent"=refnum, "Index"=0} ("Cluster"), binary string=w487, error in (no error)=w485) -> (value=w484:T14, error out=w483:errorcluster)  [unwired: 2 in, 1 out]
        n173 = Unbundle By Name(w484) -> ("node ref"=w478:T2, "new parent"=w477:T2, "Index"=w476:i32)
        n174 = call <vilib>:"MoveNode.vi"("error in"=w483, "index"=w476, "new parent"=w477, "node"=w478) -> ("error out"=w481:errorcluster)  [unwired: 7 in]
        n175 = call <vilib>:"Send Local Message.vi"("message queue in"=w479, "message name"="PopulateTree", "error in"=w481) -> ("error out"=w480:errorcluster)  [unwired: 10 in, 2 out]
      }
      frame "NodeDataChange" {
        n176 = call <vilib>:"Send Local Message.vi"("message queue in"=w492, "message name"="RefreshNode", "message value"=w494, "error in"=w495) -> ("error out"=w493:errorcluster)  [unwired: 9 in, 2 out]
        n177 = Bundle By Name(cluster=w496, "unsaved changes"=TRUE) -> (w490:T1)
      }
    }
  }
  n178 = while "User Interface Event Handler" {
    tunnel: w14 -> [w503]
    tunnel: w13 -> [w499]
    tunnel: w5 -> [w498]
    tunnel: [w497] -> w1
    stop <- w502 stop-if-true
    n179 = event shown="[2] \"View\": Shortcut Menu Selection (User)" {
      selector: w498 -> [_ _ _ _ _ _ _ _ _ _ _]
      dyn-events: [_ _ _ _ _ _ _ _ _ _ _] -> w497
      timeout: 250 -> [_ _ _ _ _ _ _ _ _ _ _]
      tunnel: w503 -> [w506 w514 w538 w588 w617 w624 w653 w658 w668 w674 w720]
      tunnel: [_ _ _ _ TRUE _ _ _ _ _ _] -> w502
      tunnel: [w506 w514 w535 w586 w613 w624 w650 w658 w666 w673 w721] -> w501
      tunnel: [w505 w510 w534 w585 w614 w620 w649 w655 w664 w671 _] -> w500
      tunnel: w499 -> [w505 w513 w533 w587 w615 w623 w648 w657 w665 w672 _]
      event Timeout {
        # "Timeout code can be added here for autosave or Lock Screen"
        n180 = event-data() -> ()  [unwired: 1 in, 1 out]
      }
      event "View": Shortcut Menu Activation? {
        n181 = event-data() -> ("CtlRef"=w520:refnum<vi>, "Coords"=w519:T19, "MenuRef"=w516:refnum<k9>)  [unwired: 1 in]
        n182 = invoke class="Tree (strict)" method="Point To Row Column"(reference=w520, error in=w513, "Point"=w519) -> (error out=w512:errorcluster, "Tag"=w518:string)  [unwired: 5 in, 6 out]
        n183 = call <vilib>:"IDtoNode.vi"("error in"=w512, "ID"=w518) -> ("error out"=w508:errorcluster, "invalid Id"=w515:bool, "node ref"=w517:T2)  [unwired: 7 in]
        n184 = case shown="False" w515 {
          tunnel: w517 -> [w525 _]
          tunnel: w516 -> [w524 _]
          tunnel: [w523 _] -> w511
          tunnel: [w522 _] -> w509
          tunnel: w508 -> [w521 w531]
          tunnel: [w521 w531] -> w507
          frame False {
            n185 = in-place {
              in-place-border: w524 -> [w528]
              in-place-border: [w526] -> w523
              n186 = in-place-dvr #7(w525) -> (w530:refnum<class "NISE_CEF_Node.lvclass">, w527:errorcluster)
              n187 = call-dynamic "ShortcutMenu.vi"("error in"=w527, "menu ref in"=w528, "node in"=w530) -> ("error out"=w526:errorcluster, "node out"=w529:refnum<class "NISE_CEF_Node.lvclass">)  [unwired: 6 in, 1 out]
              n188 = in-place-dvr #7(w529) -> (w522:errorcluster)  [unwired: 1 out]
            }
          }
          frame True {
          }
        }
        n189 = Merge Errors(w509, w511, w507) -> (w510:errorcluster)
        n190 = event-data() -> ()  [unwired: 2 in, 1 out]
      }
      event "View": Shortcut Menu Selection (User) {
        n191 = event-data() -> ("ItemPath"=w537:string, "CtlRef"=w541:refnum<vi>, "Coords"=w542:T19)  [unwired: 1 in]
        n192 = invoke class="Tree (strict)" method="Point To Row Column"(reference=w541, error in=w533, "Point"=w542) -> (error out=w532:errorcluster, "Tag"=w536:string)  [unwired: 5 in, 6 out]
        n193 = Match Pattern(string=w537, regular expression=":") -> (before substring=w540:string, after substring=w539:string)  [unwired: 1 in, 2 out]
        n194 = case shown="Default" w540 {
          selector: w540 -> [w544 _ _ _]
          tunnel: w539 -> [_ _ _ w565]
          tunnel: w538 -> [w551 w558 w564 w571]
          tunnel: w536 -> [w546 w556 w562 w570]
          tunnel: [w548 w555 w561 w568] -> w535
          tunnel: [w549 w554 w559 w566] -> w534
          tunnel: w532 -> [w550 w553 w560 w567]
          frame Default {
            n195 = Concatenate Strings(w544, ":" ("string"), w546) -> (w547:string)
            n196 = call <vilib>:"Send Local Message.vi"("message queue in"=w551, "message name"="CustomMenuAction" ("Message Name"), "message value"=w547, "error in"=w550) -> ("message queue out"=w548:T12, "error out"=w549:errorcluster)  [unwired: 9 in, 1 out]
          }
          frame "Remove" {
            n197 = call <vilib>:"Send Local Message.vi"("message queue in"=w558, "message name"="RemoveNode" ("Message Name"), "message value"=w556, "error in"=w553) -> ("message queue out"=w555:T12, "error out"=w554:errorcluster)  [unwired: 9 in, 1 out]
          }
          frame "Duplicate" {
            n198 = call <vilib>:"Send Local Message.vi"("message queue in"=w564, "message name"="Duplicate" ("Message Name"), "message value"=w562, "error in"=w560) -> ("message queue out"=w561:T12, "error out"=w559:errorcluster)  [unwired: 9 in, 1 out]
          }
          frame "Add" {
            n199 = Bundle By Name(cluster=T13 {"node type"="", "to add to"=""} ("input cluster"), "node type"=w565, "to add to"=w570) -> (w572:T13)
            n200 = Flatten To String(anything=w572) -> (data string=w573:string)  [unwired: 3 in, 2 out]
            n201 = call <vilib>:"Send Local Message.vi"("message queue in"=w571, "message name"="Add" ("Message Name"), "message value"=w573, "error in"=w567) -> ("message queue out"=w568:T12, "error out"=w566:errorcluster)  [unwired: 9 in, 1 out]
          }
        }
      }
      event "View": Drop {
        n202 = event-data() -> ("CtlRef"=w591:refnum<vi>, "Coords"=w590:T19)  [unwired: 1 in]
        n203 = invoke class="Tree (strict)" method="Point To Row Column"(reference=w591, error in=w587, "Point"=w590) -> (reference out=w589:refnum<vi>, error out=w584:errorcluster, "Tag"=w581:string)  [unwired: 5 in, 5 out]
        n204 = call <vilib>:"ValidDragDrop.vi"("error in"=w584, "Reorder"=TRUE, "drag over"=w581, "Tree Ref in"=w589) -> ("Error Out"=w576:errorcluster, "Accepted"=w579:bool, "Drag"=w583:string, "Tree Ref out"=w593:refnum<vi>, "Moved Node"=w577:T2, "Position"=w575:i32, "Parent Node"=w578:T2, "Parent"=w580:string)
        n205 = case shown="False" w579 {
          tunnel: w583 -> [_ w610]
          tunnel: w593 -> [_ w612]
          tunnel: [_ TRUE] -> w592
          tunnel: w580 -> [_ w608]
          tunnel: w588 -> [w595 w607]
          tunnel: [w595 w603] -> w586
          tunnel: [w594 w602] -> w585
          tunnel: w577 -> [_ w598]
          tunnel: w578 -> [_ w597]
          tunnel: w576 -> [w594 w599]
          tunnel: w575 -> [_ w596]
          frame False {
          }
          frame True {
            n206 = invoke class="Tree (strict)" method="Edit Tree Items.Move Item"(reference=w612, error in=w599, "tag"=w610, "New Parent"=w608) -> (error out=w600:errorcluster)  [unwired: 3 in, 6 out]
            n207 = Bundle By Name(cluster=T14 {"node ref"=refnum, "new parent"=refnum, "Index"=0} ("Cluster"), "Index"=w596, "node ref"=w598, "new parent"=w597) -> (w606:T14)
            n208 = Flatten To String(anything=w606, error in (no error)=w600) -> (data string=w605:string, error out=w601:errorcluster)  [unwired: 2 in, 1 out]
            n209 = call <vilib>:"Send Local Message.vi"("message queue in"=w607, "message name"="Move", "message value"=w605, "error in"=w601) -> ("message queue out"=w603:T12, "error out"=w602:errorcluster)  [unwired: 9 in, 1 out]
          }
        }
        n210 = event-data("Accepted?"=w592) -> ()  [unwired: 1 in, 1 out]
      }
      event "Exit": Value Change {
        # "Exit the application                                           >> Stop this message generator loop    Cleaning errors if the other loop stop this one"
        n211 = event-data() -> ()  [unwired: 1 in, 1 out]
        n212 = call <vilib>:"Send Local Message.vi"("message queue in"=w617, "message name"="Close", "error in"=w615) -> ("message queue out"=w613:T12, "error out"=w618:errorcluster)  [unwired: 10 in, 1 out]
        n213 = call <vilib>:"Clear Errors.vi"("error in (no error)"=w618) -> ("error out"=w614:errorcluster)  [unwired: 5 in, 1 out]
      }
      event "View": Drag Starting? {
        n214 = event-data() -> ("Data"=w630:T20, "CtlRef"=w632:refnum<vi>, "Coords"=w631:T19)  [unwired: 1 in]
        n215 = invoke class="Tree (strict)" method="Point To Row Column"(reference=w632, error in=w623, "Point"=w631) -> (error out=w622:errorcluster, "Tag"=w629:string)  [unwired: 5 in, 6 out]
        n216 = call <vilib>:"IDtoNode.vi"("error in"=w622, "ID"=w629) -> ("error out"=w621:errorcluster, "invalid Id"=w628:bool, "node ref"=w627:T2)  [unwired: 7 in]
        n217 = case shown="False" w628 {
          tunnel: w627 -> [w640 _]
          tunnel: [w637 TRUE ("Removable")] -> w625
          tunnel: w621 -> [w636 w646]
          tunnel: [w633 w646] -> w620
          frame False {
            n218 = in-place {
              in-place-border: [w643] -> w639
              in-place-border: w636 -> [w642]
              in-place-border: [w641] -> w635
              n219 = in-place-dvr #8(w640) -> (w645:refnum<class "NISE_CEF_Node.lvclass">)  [unwired: 1 out]
              n220 = call-dynamic "EditOptions.vi"("error in"=w642, "node in"=w645) -> ("error out"=w641:errorcluster, "edit options"=w643:T21, "node out"=w644:refnum<class "NISE_CEF_Node.lvclass">)  [unwired: 6 in, 1 out]
              n221 = in-place-dvr #8(w644) -> (w634:errorcluster)  [unwired: 1 out]
            }
            n222 = Unbundle By Name(w639) -> ("movable"=w638:bool)
            n223 = Merge Errors(w634, w635) -> (w633:errorcluster)
            n224 = Not(x=w638) -> (.not. x?=w637:bool)
          }
          frame True {
          }
        }
        n225 = event-data("Data"=w630, "Drag Mode"=enum32{"copy or move", "copy only", "move only"}."move only", "Discard?"=w625) -> ()  [unwired: 1 in, 1 out]
      }
      event "View": Value Change {
        n226 = event-data() -> ("NewVal"=w651:string)  [unwired: 1 in]
        n227 = call <vilib>:"Send Local Message.vi"("message queue in"=w653, "message name"="ActivateNode" ("Message Name"), "message value"=w651, "error in"=w648) -> ("message queue out"=w650:T12, "error out"=w649:errorcluster)  [unwired: 9 in, 1 out]
      }
      event "View": event type 3.0.xa000003a {
        n228 = event-data() -> ("CtlRef"=w663:refnum<vi>, "Coords"=w660:T19)  [unwired: 1 in]
        n229 = invoke class="Tree (strict)" method="Point To Row Column"(reference=w663, error in=w657, "Point"=w660) -> (reference out=w662:refnum<vi>, error out=w656:errorcluster, "Tag"=w661:string)  [unwired: 5 in, 5 out]
        n230 = call <vilib>:"ValidDragDrop.vi"("error in"=w656, "Reorder"=TRUE, "drag over"=w661, "Tree Ref in"=w662) -> ("Error Out"=w655:errorcluster, "Accepted"=w659:bool)  [unwired: 6 out]
        n231 = event-data("Accepted?"=w659) -> ()  [unwired: 1 in, 1 out]
      }
      event Panel Close? {
        # "Intercepts the upper right close panel operation to allow a smooth shutdown as opposed to immediately killing the app."
        n232 = event-data() -> ()  [unwired: 1 in, 1 out]
        n233 = call <vilib>:"Send Local Message.vi"("message queue in"=w668, "message name"="Close?", "error in"=w665) -> ("message queue out"=w666:T12, "error out"=w664:errorcluster)  [unwired: 10 in, 1 out]
        n234 = event-data("Discard?"=TRUE) -> ()  [unwired: 1 in, 1 out]
      }
      event Menu Selection (User) {
        # "#USERCFG It is needed to add a Case for Every item on the menu"
        n235 = event-data() -> ("ItemTag"=w670:string, "ItemPath"=w675:string)  [unwired: 1 in]
        n236 = case shown="\"_Tools:Multiple Parameter Editor\"" w675 {
          selector: w675 -> [w679 _ _ _ _ _ _]
          tunnel: w674 -> [w684 w689 w694 w699 w704 w709 w718]
          tunnel: [w684 w685 w690 w695 w700 w705 w715] -> w673
          tunnel: w672 -> [w681 w687 w692 w697 w702 w707 w714]
          tunnel: [w680 w686 w691 w696 w701 w706 w712] -> w671
          tunnel: w670 -> [w678 _ _ _ _ _ _]
          frame Default {
            n237 = Concatenate Strings(w678, "::" ("string"), w679) -> (w677:string)
            n238 = call <vilib>:"NISE_error generator.vi"("error in"=w681, "source"="configuration tool main.vi", "append error message"=w677, "error code (0)"=538506) -> ("error out"=w680:errorcluster)  [unwired: 5 in]
          }
          frame "_File:_New" {
            n239 = call <vilib>:"Send Local Message.vi"("message queue in"=w689, "message name"="New?" ("Message Name"), "error in"=w687) -> ("message queue out"=w685:T12, "error out"=w686:errorcluster)  [unwired: 10 in, 1 out]
          }
          frame "_File:_Open" {
            n240 = call <vilib>:"Send Local Message.vi"("message queue in"=w694, "message name"="Open?" ("Message Name"), "error in"=w692) -> ("message queue out"=w690:T12, "error out"=w691:errorcluster)  [unwired: 10 in, 1 out]
          }
          frame "_File:_Save" {
            n241 = call <vilib>:"Send Local Message.vi"("message queue in"=w699, "message name"="Save" ("Message Name"), "error in"=w697) -> ("message queue out"=w695:T12, "error out"=w696:errorcluster)  [unwired: 10 in, 1 out]
          }
          frame "_File:Save As..." {
            n242 = call <vilib>:"Send Local Message.vi"("message queue in"=w704, "message name"="SaveAs" ("Message Name"), "error in"=w702) -> ("message queue out"=w700:T12, "error out"=w701:errorcluster)  [unwired: 10 in, 1 out]
          }
          frame "_File:_Exit" {
            n243 = call <vilib>:"Send Local Message.vi"("message queue in"=w709, "message name"="Close?" ("Message Name"), "error in"=w707) -> ("message queue out"=w705:T12, "error out"=w706:errorcluster)  [unwired: 10 in, 1 out]
          }
          frame "_Tools:Multiple Parameter Editor" {
            n244 = call <vilib>:"Send Local Message.vi"("message queue in"=w718, "message name"="CleansubPanel", "error in"=w714) -> ("message queue out"=w717:T12, "error out"=w713:errorcluster)  [unwired: 10 in, 1 out]
            n245 = call <vilib>:"Send Local Message.vi"("message queue in"=w717, "message name"="Custom View" ("Message Name"), "message value"="Multiple Variable Editor" ("Message Name"), "error in"=w713) -> ("message queue out"=w715:T12, "error out"=w712:errorcluster)  [unwired: 9 in, 1 out]
          }
        }
      }
      event User Event {
        n246 = event-data() -> ("node ref"=w719:T2)  [unwired: 1 in]
        n247 = call <vilib>:"NodetoID.vi"("node ref"=w719) -> ("ID"=w722:string)  [unwired: 9 in, 1 out]
        n248 = call <vilib>:"Send Local Message.vi"("message queue in"=w720, "message name"="NodeDataChange", "message value"=w722) -> ("message queue out"=w721:T12)  [unwired: 10 in, 2 out]
      }
    }
    n249 = call "Error.vi"("error in (no error)"=w500, "message queue in"=w501) -> ()  [unwired: 9 in, 1 out]
  }
  n250 = Unregister For Events(event registration refnum=w1) -> (error out=w2:errorcluster)  [unwired: 1 in]
  n251 = Merge Errors(w2, w7) -> (w3:errorcluster)
  n252 = call <vilib>:"DestroyStandardEvents.vi"("error in"=w3, "standard events"=w6) -> ()  [unwired: 9 in, 1 out]
